vi "Is Steady State.vi"(11 "Angle":dbl[unit]) -> (3 "Settled":bool)   [LabVIEW 2020]
uses:
  <vilib>/ptbypt/NI_PtbyPt.lvlib
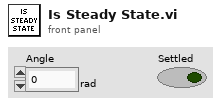
[diagram p1: front panel]
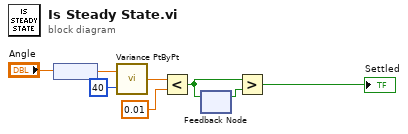
[diagram p0: block diagram]
diagram:
  n1 = node("Angle") -> (w4:dbl)
  n2 = call <vilib>:"Variance PtByPt.vi"("x"=w4, "sample length"=40) -> ("variance"=w3:dbl)  [unwired: 1 in, 2 out]
  n3 = Less?(x=w3, y=0.01) -> (x < y?=w1:bool)
  n4 = feedback #1() -> (w2:bool)  [unwired: 1 in]
  n5 = feedback-in #1(w1) -> ()
  n6 = Greater?(x=w1, y=w2) -> (0:→"Settled":bool)
